vi "X Button.vi"(8 "error in":errorcluster) -> (0 "error out":errorcluster, 3 "constants cluster":cluster{"a":dbl, "b":dbl, "c":dbl, "d":dbl})   [LabVIEW 2017, in "Huskie Swerve.lvlib"]
uses:
  Huskie Swerve.lvlib
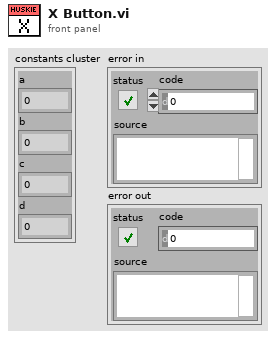
[diagram p1: front panel]
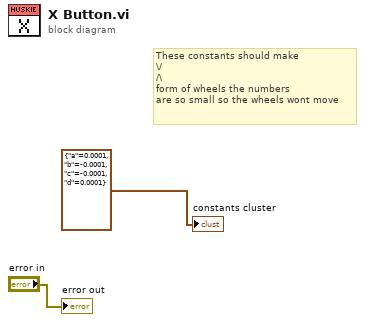
[diagram p0: block diagram]
diagram:
  # "These constants should make \n\\/\n/\\\nform of wheels the numbers \nare so small so the wheels wont move"
  "constants cluster" <- cluster{"a":dbl, "b":dbl, "c":dbl, "d":dbl} {"a"=0.0001, "b"=-0.0001, "c"=-0.0001, "d"=0.0001} ("constants cluster 2")
  "error out" <- "error in"
